vi "SysInfo-Version String.vi"() -> (0 "Version String":string)   [LabVIEW 2020]
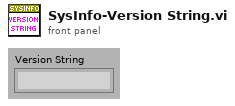
[diagram p1: front panel]
types:
  T1 = cluster{"Major":i32, "Minor":i32, "Build":i32, "Private":i32, "FileVersion":string, "ProductName":string, "InternalName":string, "CompanyName":string, "LegalCopyright":string, "FileDescription":string}
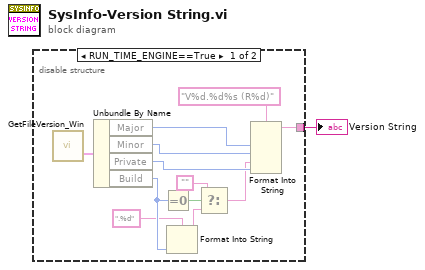
[diagram p0: block diagram]
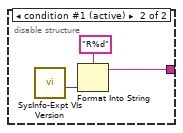
[diagram p2: hidden frame]
diagram:
  n1 = disable-structure shown="RUN_TIME_ENGINE==True" {
    disable-tunnel: [w11 w14] -> w1
    frame condition #0 {
      n2 = call "GetFileVersion_Win.vi"() -> ("File Info Out"=w12:T1)  [unwired: 9 in, 2 out]
      n3 = Unbundle By Name(w12) -> ("Major"=w10:i32, "Minor"=w9:i32, "Private"=w8:i32, "Build"=w5:i32)
      n4 = Equal To 0?(x=w5) -> (x = 0?=w7:bool)
      n5 = Format Into String(format string=".%d", w5) -> (resulting string=w3:string)  [unwired: 2 in, 1 out]
      n6 = Select(t="", s=w7, f=w3) -> (s? t:f=w2:string)
      n7 = Format Into String(format string="V%d.%d%s (R%d)", w10, w9, w2, w8) -> (resulting string=w11:string)  [unwired: 2 in, 1 out]
    }
    frame condition #1 (active) {
      n8 = call "SysInfo-Expt VIs Version.vi"() -> ("Expt VIs Version out"=w15:i32)  [unwired: 11 in]
      n9 = Format Into String(format string="R%d" ("PF Version"), w15) -> (resulting string=w14:string)  [unwired: 2 in, 1 out]
    }
  }
  "Version String" <- w1
